vi "Verify Basic Information.vi"(8 "에러 입력(에러 없음)":errorcluster, 10 "교정정보 in":T1, 11 "교정정보 in":refnum<vi>) -> (0 "에러 출력":errorcluster, 2 "문자열":string, 3 "OK?":bool)   [LabVIEW 2020]
uses:
  Controls/Clst_Cal Info Global.ctl
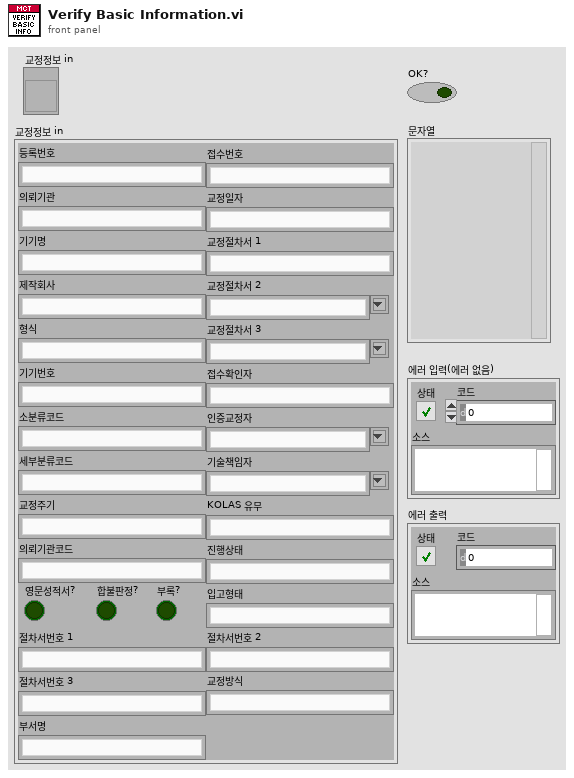
[diagram p1: front panel]
types:
  T1 = typedef "Clst_Cal Info Global.ctl" = cluster{"등록번호":string, "의뢰기관":string, "기기명":string, "제작회사":string, "형식":string, "기기번호":string, "소분류코드":string, "세부분류코드":string, "교정주기":string, "접수번호":string, "교정일자":string, "교정절차서 1":string, "교정절차서 2":string, "교정절차서 3":string, "접수확인자":string, "인증교정자":string, "기술책임자":string, "KOLAS 유무":string, "진행상태":string, "의뢰기관코드":string, "입고형태":string, "영문성적서?":bool, "합불판정?":bool, "부록?":bool, "절차서번호 1":string, "절차서번호 2":string, "절차서번호 3":string, "교정방식":string, "부서명":string}
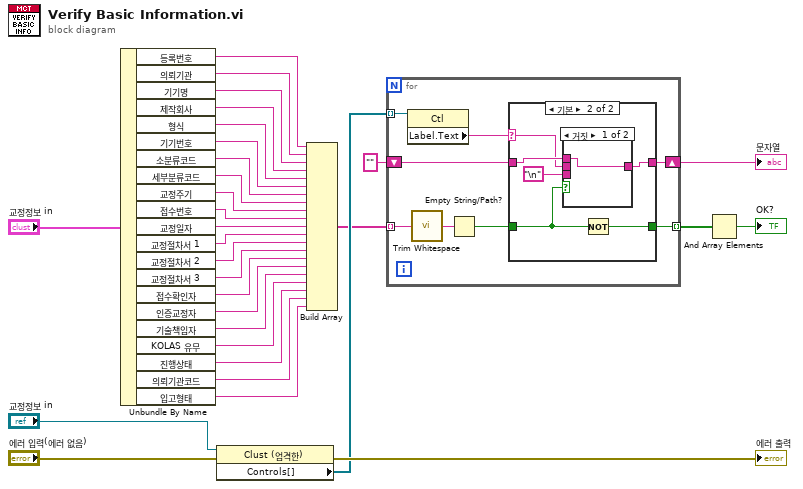
[diagram p0: block diagram]
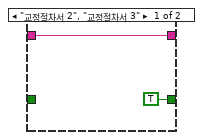
[diagram p2: hidden frame]
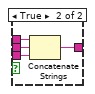
[diagram p3: hidden frame]
diagram:
  n1 = Unbundle By Name("교정정보 in") -> ("등록번호"=w2:string, "의뢰기관"=w3:string, "기기명"=w4:string, "제작회사"=w5:string, "형식"=w6:string, "기기번호"=w7:string, "소분류코드"=w8:string, "세부분류코드"=w9:string, "교정주기"=w10:string, "접수번호"=w11:string, "교정일자"=w12:string, "교정절차서 1"=w13:string, "교정절차서 2"=w14:string, "교정절차서 3"=w15:string, "접수확인자"=w16:string, "인증교정자"=w17:string, "기술책임자"=w18:string, "KOLAS 유무"=w19:string, "진행상태"=w20:string, "의뢰기관코드"=w21:string, "입고형태"=w22:string)
  n2 = property class="Clust (엄격한)"(reference="교정정보 in", error in="에러 입력(에러 없음)") -> (error out=→"에러 출력":errorcluster, "Controls[]"=w24:refnum<vi>[])  [unwired: 1 out]
  n3 = Build Array(w2, w3, w4, w5, w6, w7, w8, w9, w10, w11, w12, w13, w14, w15, w16, w17, w18, w19, w20, w21, w22) -> (w23:string[])
  n4 = for {
    tunnel: w23 -> [w38] mode=indexing
    tunnel: w24 -> [w39] mode=indexing
    shift-right: [w36] -> w25
    shift-left: "" -> [w35]
    tunnel: [w33] -> w26 mode=indexing
    n5 = property class="Ctl"(reference=w39) -> ("Label.Text"=w32:string)  [unwired: 1 in, 2 out]
    n6 = call <vilib>:"Trim Whitespace.vi"("string"=w38) -> ("trimmed string"=w37:string)  [unwired: 1 in]
    n7 = Empty String/Path?(string/path=w37) -> (empty?=w34:bool)
    n8 = case shown="기본" w32 {
      selector: w32 -> [_ w42]
      tunnel: [w41 w47] -> w36
      tunnel: w35 -> [w41 w46]
      tunnel: w34 -> [_ w44]
      tunnel: [TRUE w43] -> w33
      frame "교정절차서 2", "교정절차서 3" {
      }
      frame Default {
        n9 = case shown="거짓" w44 {
          tunnel: [w48 w52] -> w47
          tunnel: w46 -> [w48 w51]
          tunnel: w42 -> [_ w50]
          tunnel: "\n" -> [_ w49]
          frame False {
          }
          frame True {
            n10 = Concatenate Strings(w51, w50, w49) -> (w52:string)
          }
        }
        n11 = Not(x=w44) -> (.not. x?=w43:bool)
      }
    }
  }
  "문자열" <- w25
  n12 = And Array Elements(Boolean array=w26) -> (logical AND=→"OK?":bool)
